vi "WebCam.Example03.vi"() -> ()   [LabVIEW 2011]
panel:
  in  "Case Constant\n(See Context Help)":bool
  in  "stop":bool
  out "error out":errorcluster
  in  "error in (no error)":errorcluster
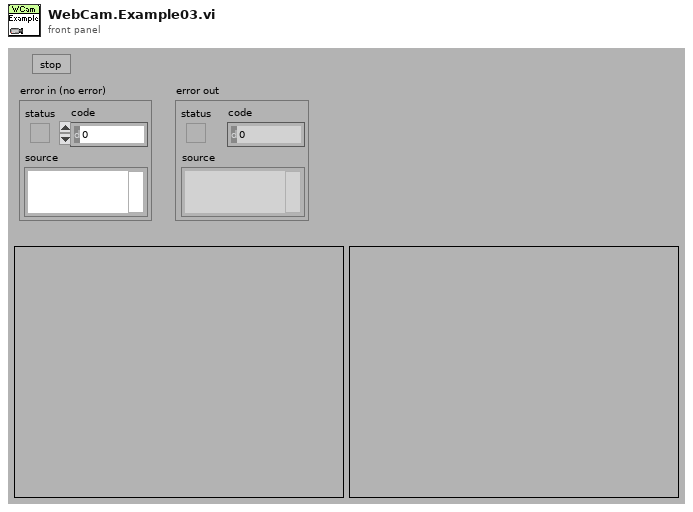
[diagram p1: front panel]
types:
  T1 = cluster{"posX":i32, "posY":i32, "nWidth":i32, "nHeight":i32}
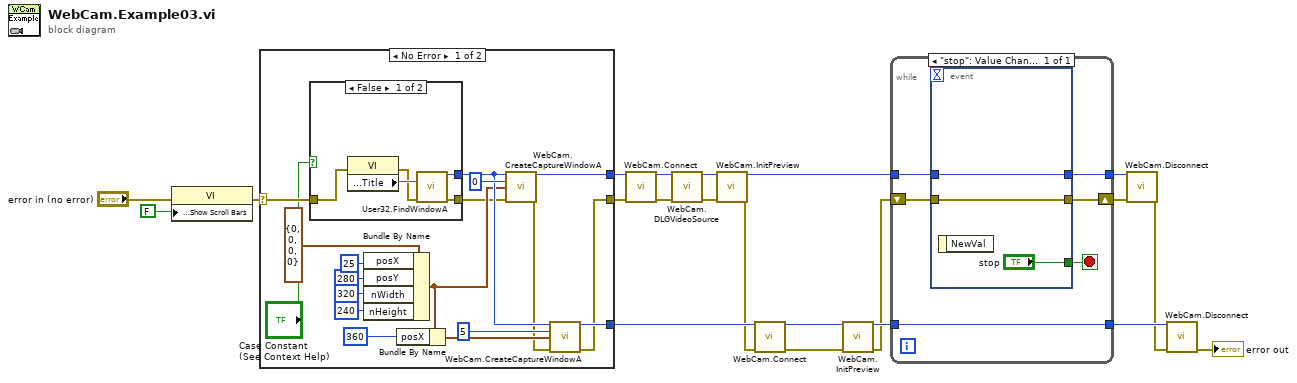
[diagram p0: block diagram]
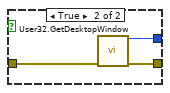
[diagram p2: hidden frame]
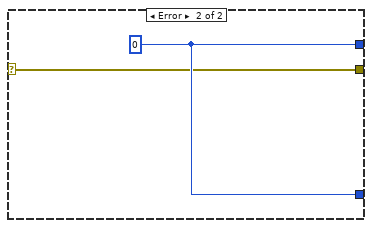
[diagram p3: hidden frame]
diagram:
  n1 = property class="VI"(error in="error in (no error)", "Front Panel Window:Show Scroll Bars"=FALSE) -> (error out=w17:errorcluster)  [unwired: 1 in, 1 out]
  n2 = case shown="No Error" w17 {
    selector: w17 -> [w38 w48]
    tunnel: [w39 w49] -> w11
    tunnel: [w22 w48] -> w10
    tunnel: [w28 w49] -> w15
    frame No Error {
      n3 = case shown="False" "Case Constant\n(See Context Help)" {
        tunnel: w38 -> [w41 w47]
        tunnel: [w44 w46] -> w31
        tunnel: [w43 w45] -> w23
        frame False {
          n4 = property class="VI"(error in=w41) -> (error out=w40:errorcluster, "Front Panel Window:Title"=w42:string)  [unwired: 1 in, 1 out]
          n5 = call "User32.FindWindowA.vi"("lpWindowName"=w42, "error in (no error)"=w40) -> ("hwnd"=w44:i32, "error out"=w43:errorcluster)  [unwired: 12 in]
        }
        frame True {
          n6 = call "User32.GetDesktopWindow.vi"("error in (no error)"=w47) -> ("Desktop handle"=w46:i32, "error out"=w45:errorcluster)  [unwired: 13 in]
        }
      }
      n7 = Bundle By Name(cluster=T1 {"posX"=0, "posY"=0, "nWidth"=0, "nHeight"=0} ("rect"), "posX"=25 ("nWidth"), "posY"=280 ("nWidth"), "nWidth"=320, "nHeight"=240 ("nWidth")) -> (w29:T1)
      n8 = Bundle By Name(cluster=w29, "posX"=360) -> (w26:T1)
      n9 = call "WebCam.CreateCaptureWindowA.vi"("handle"=w31, "nID"=0, "rect"=w29, "error in (no error)"=w23) -> ("handle out"=w39:i32, "error out"=w24:errorcluster)  [unwired: 10 in]
      n10 = call "WebCam.CreateCaptureWindowA.vi"("handle"=w31, "nID"=5, "rect"=w26, "error in (no error)"=w24) -> ("handle out"=w28:i32, "error out"=w22:errorcluster)  [unwired: 10 in]
    }
    frame Error {
      w49 = 0
    }
  }
  n11 = call "WebCam.Connect.vi"("handle"=w11, "error in (no error)"=w10) -> ("handle out"=w8:i32, "error out"=w7:errorcluster)  [unwired: 12 in]
  n12 = call "WebCam.DLGVideoSource.vi"("handle"=w8, "error in (no error)"=w7) -> ("handle out"=w5:i32, "error out"=w6:errorcluster)  [unwired: 12 in]
  n13 = call "WebCam.InitPreview.vi"("handle"=w5, "error in (no error)"=w6) -> ("handle out"=w20:i32, "error out"=w4:errorcluster)  [unwired: 12 in]
  n14 = call "WebCam.Connect.vi"("handle"=w15, "error in (no error)"=w4) -> ("handle out"=w2:i32, "error out"=w1:errorcluster)  [unwired: 12 in]
  n15 = call "WebCam.InitPreview.vi"("handle"=w2, "error in (no error)"=w1) -> ("handle out"=w14:i32, "error out"=w3:errorcluster)  [unwired: 12 in]
  n16 = while {
    shift-right: [w55] -> w21
    shift-left: w3 -> [w54]
    tunnel: w20 -> [w52]
    tunnel: [w51] -> w19
    tunnel: w14 -> [w50]
    tunnel: [w50] -> w13
    stop <- w53 stop-if-true
    n17 = event shown="[0] \"stop\": Value Change" {
      selector: _ -> [_]
      dyn-events: _ -> [_]
      timeout: _ -> [_]
      tunnel: [w58] -> w55
      tunnel: w54 -> [w58]
      tunnel: ["stop"] -> w53
      tunnel: w52 -> [w56]
      tunnel: [w56] -> w51
      event "stop": Value Change {
        n18 = event-data() -> ()  [unwired: 1 in, 1 out]
      }
    }
  }
  n19 = call "WebCam.Disconnect.vi"("handle"=w19, "error in (no error)"=w21) -> ("error out"=w12:errorcluster)  [unwired: 13 in]
  n20 = call "WebCam.Disconnect.vi"("handle"=w13, "error in (no error)"=w12) -> ("error out"=→"error out":errorcluster)  [unwired: 13 in]
